vi "Experiment header-Generate missing stats.vi"(11 "Experiment folder path":path) -> (3 "STATS array":dbl[](array[numeric]))   [LabVIEW 2013]
uses:
  Typedefs/Test header stats cluster.ctl
  Typedefs/Logging queue element.ctl
  Typedefs/Imaging Protocols enum.ctl
  Typedefs/Frame Size.ctl
  Typedefs/Acquired points count.ctl
  Typedefs/Save-Load-Save as-Load last enum.ctl
  Typedefs/Header file type enum.ctl
panel:
  out "STATS cluster":T1
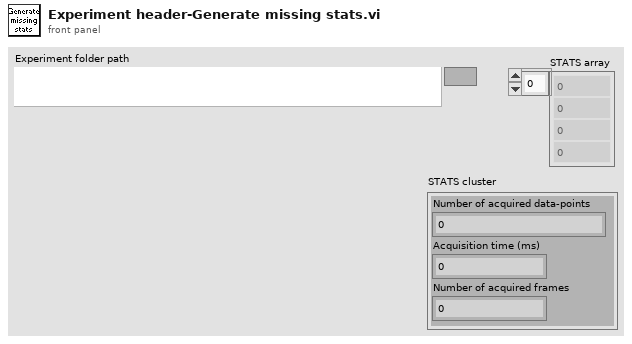
[diagram p1: front panel]
types:
  T1 = typedef "Test header stats cluster.ctl" = cluster{"Number of acquired data-points":dbl, "Acquisition time (ms)":dbl, "Number of acquired frames":dbl}
  T2 = typedef "Imaging Protocols enum.ctl" = enum16{"AOL Z-Stack", "Motor Z Stack", "Functional Acquisition", "Single Plane Acquisition", "Volume Acquisition", "Live Imaging", "Live Plane Imaging", "Live Volume Imaging"}
  T3 = typedef "Header file type enum.ctl" = enum16{"All parameters", "Params for funct acq w ROI or mscn", "Params for funct acq w rectangles", "Live imaging header parameters", "AOL Parameters"}
  T4 = typedef "Save-Load-Save as-Load last enum.ctl" = enum16{"Save file", "Save file as", "Load file", "Load last file"}
  T5 = typedef "Logging queue element.ctl" = cluster{"Imaging Protocol":T2, "Number of Trials":u16, "Frame Size":T6, "# Averaged frames":u16, "Dwell time (us)":dbl, "Index of Z-plane":i32, "Timelapse?":bool, "Logging process is active":bool, "Speed logging enabled":bool, "tdms file ref":refnum<k34>, "path":path, "Trial Number":i32, "Expected # points acquired":bool, "Manually stopped":bool, "Ch0 data":u32[], "Ch1 data":u32[], "Last trial":bool, "Points acquired":T7}
  T6 = typedef "Frame Size.ctl" = u16
  T7 = typedef "Acquired points count.ctl" = cluster{"Ch0 last trial":u64, "Ch1 last trial":u64, "All trials":u64}
  T8 = typedef "Header parameters cluster-ALL.ctl" = cluster{"Imaging Protocol":T2, "Number of POI":u16, "Number of Miniscans":u16, "Number of Trials":u16, "Number of Cycles ":u64, "# Averaged Frames":u16, "Laser power (%)":u8, "Pockels":dbl, "Acquisition Length (sec)":dbl, "Fill time (us)":dbl, "POI Dwell time (us)":dbl, "Miniscan Dwell time per pixel (us)":dbl, "PMT 1":dbl, "PMT 2":dbl, "Back Apperture":dbl, "Zoom":dbl, "Frame Size":T6, "Center Frequency":dbl, "Field of View":dbl, "DwellTime (us)":dbl, "Wavelength (nm)":dbl, "AOL Z":dbl, "AOL Mode":T9, "GridXY":dbl, "GridZ":dbl, "TriggerDelay (sec)":dbl, "Number of Pixels in Miniscan":u16, "Experiment folder path":path, "X centre":dbl, "Y centre":dbl, "Angle (degrees)":dbl, "Plane Mode":T10, "Software version":dbl, "Objective":T11, "MotorZ Calibration":u32, "Pockels Calibration":u32, "Threshold":u16[], "Video length (sec)":dbl, "Frame rate (fps)":u8, "Rectangle ROI length (pixels)":u16, "Rectangle ROI height (pixels)":u16}
  T9 = typedef "AOL modes.ctl" = enum16{"Raster", "Structural", "Pointing", "Mini Scan", "Alignment"}
  T10 = typedef "Plane Mode.ctl" = u16
  T11 = typedef "Objective selector control enum.ctl" = string
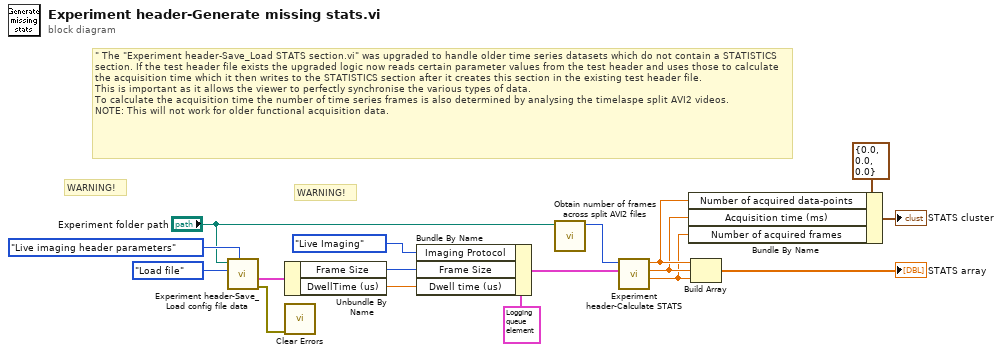
[diagram p0: block diagram]
diagram:
  # "WARNING!"
  # "WARNING!"
  # "\"\tThe \"Experiment header-Save_Load STATS section.vi\" was upgraded to handle older time series datasets which do not contain a STATISTICS section. If the test header file exists the upgraded logic now reads certain parameter values from the test header and uses those to calculate the acquisition time which it then writes to the STATISTICS section after it creates this section in the existing test header file. \nThis is important as it allows the viewer to perfectly synchronise the various types of data.\nTo calculate the acquisition time the number of time series frames is also determined by analysing the timelaspe split AVI2 videos. \nNOTE: This will not work for older functional acquisition data."
  n1 = call "Experiment header-Save_Load config file data.vi"("Header file type"=Header_file_type_enum."Live imaging header parameters", "Function"=Save-Load-Save_as-Load_last_enum."Load file", "Experiment data folder path"="Experiment folder path") -> ("error out"=w10:errorcluster, "All header parameters out"=w9:T8)  [unwired: 7 in]
  n2 = Unbundle By Name(w9) -> ("Frame Size"=w12:T6, "DwellTime (us)"=w11:dbl)
  n3 = call <vilib>:"Clear Errors.vi"("error in (no error)"=w10) -> ()  [unwired: 6 in, 1 out]
  n4 = Bundle By Name(cluster=T5 {"Imaging Protocol"=enum."Live Imaging", "Number of Trials"=0, "Frame Size"=0, "# Averaged frames"=0, "Dwell time (us)"=0.1, "Index of Z-plane"=0, "Timelapse?"=FALSE, "Logging process is active"=FALSE, "Speed logging enabled"=FALSE, "tdms file ref"=refnum, "path"=path "", "Trial Number"=0, "Expected # points acquired"=FALSE, "Manually stopped"=FALSE, "Ch0 data"=[], "Ch1 data"=[], "Last trial"=FALSE, "Points acquired"={"Ch0 last trial"=0, "Ch1 last trial"=0, "All trials"=0}} ("Logging queue element"), "Imaging Protocol"=Imaging_Protocols_enum."Live Imaging", "Frame Size"=w12, "Dwell time (us)"=w11) -> (w16:T5)
  n5 = call "Obtain number of frames across split AVI2 files.vi"("Experiment folder path"="Experiment folder path") -> ("Number of Frames (across all split videos of a single channel)"=w7:u32)  [unwired: 9 in, 1 out]
  n6 = call "Experiment header-Calculate STATS.vi"("Logging queue element"=w16, "Timelapse frames saved"=w7) -> ("Number of acquired frames"=w2:dbl, "Acquisition time (ms)"=w3:dbl, "Total number of points acquired (Ch0)"=w4:dbl)  [unwired: 7 in]
  n7 = Bundle By Name(cluster=T1 {"Number of acquired data-points"=0.0, "Acquisition time (ms)"=0.0, "Number of acquired frames"=0.0} ("Read values 2"), "Number of acquired data-points"=w4, "Acquisition time (ms)"=w3, "Number of acquired frames"=w2) -> (→"STATS cluster":T1)
  n8 = Build Array(w4, w3, w2) -> (→"STATS array":dbl[])
